vi "Target Troubleshoot streams.vi"() -> ()   [LabVIEW 2018]
panel:
  out "error out":errorcluster
  out "data out":dbl
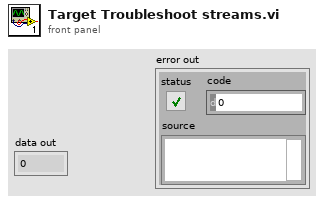
[diagram p1: front panel]
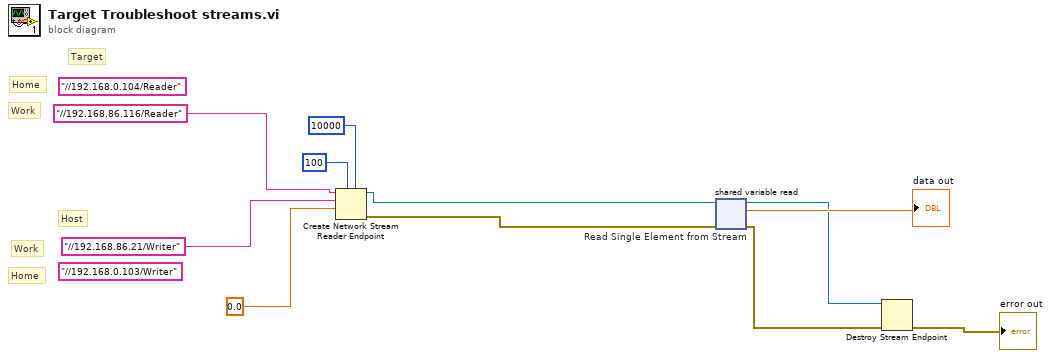
[diagram p0: block diagram]
diagram:
  (unwired) "//192.168.0.103/Writer" ("writer name")
  (unwired) "//192.168.0.104/Reader" ("reader url")
  # "Work"
  # "Home"
  # "Work"
  # "Home"
  # "Host"
  # "Target"
  n1 = Create Network Stream Reader Endpoint(5:10000 ("timeout in ms (-1)"), 7:100 ("reader buffer size"), 9:0.0, 10:"//192.168.86.21/Writer" ("writer name"), 11:"//192.168.86.116/Reader" ("reader url")) -> (0:w4:errorcluster, 3:w6:refnum<k21>)  [unwired: 2 in]
  n2 = shared-variable-read "Read Single Element from Stream"(w6, w4) -> (w3:refnum<k21>, w2:errorcluster, →"data out":dbl)  [unwired: 1 in, 1 out]
  n3 = Destroy Stream Endpoint(8:w2, 11:w3) -> (0:→"error out":errorcluster)
